vi "Stop Core.vi"(10 "final error code":i32, 11 "Nested in":refnum<class "[MV] Key Certify.lvclass">) -> (3 "Nested out":refnum<class "[MV] Key Certify.lvclass">)   [LabVIEW 2020, in "[MV] Key Certify.lvlib" / "[MV] Key Certify.lvclass"]
doc: "(<B>Filename</B>: Actor Framework.lvlib:Actor.lvclass:Stop Core.vi)\n\nDefines what the actor does before it stops. Use the <B>final error code</B> input to determine whether the actor shut down in response to an error.\n\nBy default, this method does nothing. A descendant class may override it to define behavior, such as shutting down any processes the actor initiated in its override of the Actor Core method."
uses:
  [MV] Key Certify.lvclass
  <vilib>/ActorFramework/Actor/Actor.lvclass
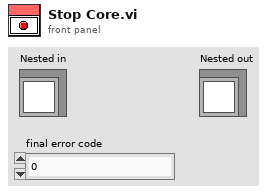
[diagram p1: front panel]
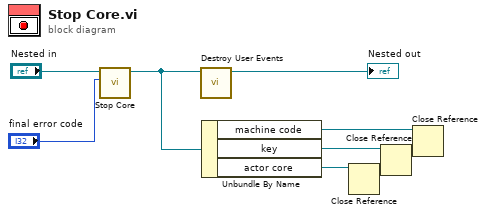
[diagram p0: block diagram]
diagram:
  n1 = call-parent "Stop Core.vi"("final error code"="final error code", "Actor in"="Nested in") -> ("Actor out"=w4:refnum<class "[MV] Key Certify.lvclass">)  [unwired: 9 in]
  n2 = call "Destroy User Events.vi"("UI Template in"=w4) -> ("UI Template out"=→"Nested out":refnum<class "[MV] Key Certify.lvclass">)  [unwired: 10 in]
  n3 = Unbundle By Name(w4) -> ("machine code"=w1:refnum<vi>, "key"=w2:refnum<vi>, "actor core"=w3:refnum<vi>)
  n4 = Close Reference(reference=w3) -> ()  [unwired: 1 in, 1 out]
  n5 = Close Reference(reference=w2) -> ()  [unwired: 1 in, 1 out]
  n6 = Close Reference(reference=w1) -> ()  [unwired: 1 in, 1 out]
